vi "CRYProject Editor PIC Open New Project.vi"   [LabVIEW 2013]
uses:
  CRYStepSetup/CRYStepSetup Global.vi
  CRYProject Editor Global.vi
types:
  T1 = cluster{"EventName":string, "Arg1":string, "Numeric":u16, "Numeric 2":u16, "AddSteps ":refnum<vi>, "Arg1 2":string, "Arg1 3":string, "Boolean":bool}
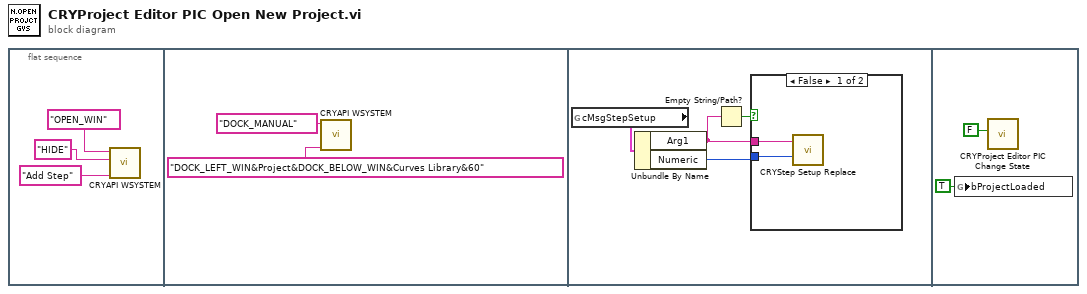
[diagram p0: block diagram]
diagram:
  n1 = flat-sequence {
    frame #0 {
      n2 = call "CRYAPI WSYSTEM.vi"("sData"="Add Step", "sOption"="HIDE" ("sAction"), "sAction"="OPEN_WIN") -> ()  [unwired: 1 in, 8 out]
    }
    frame #1 {
      n3 = call "CRYAPI WSYSTEM.vi"("sData"="DOCK_LEFT_WIN&Project&DOCK_BELOW_WIN&Curves Library&60" ("sAction"), "sAction"="DOCK_MANUAL") -> ()  [unwired: 2 in, 8 out]
    }
    frame #2 {
      n4 = global read "CRYStepSetup Global.vi" "cMsgStepSetup"() -> (w6:T1)
      n5 = Unbundle By Name(w6) -> ("Arg1"=w8:string, "Numeric"=w9:u16)
      n6 = Empty String/Path?(string/path=w8) -> (empty?=w7:bool)
      n7 = case shown="False" w7 {
        tunnel: w8 -> [w11 _]
        tunnel: w9 -> [w10 _]
        frame False {
          n8 = call "CRYStep Setup Replace.vi"("Current Step Setup VI No"=w10, "Category"=w11) -> ()  [unwired: 2 in, 8 out]
        }
        frame True {
          # "??????????/"
        }
      }
    }
    frame #3 {
      n9 = global write "CRYProject Editor Global.vi" "bProjectLoaded"(TRUE ("Project Exist?")) -> ()
      n10 = call "CRYProject Editor PIC Change State.vi"("bChangeState"=FALSE) -> ()  [unwired: 11 in]
    }
  }
